vi "pre_scan_thg.vi"(6 "scan_values":dbl[](array[numeric]), 7 "override":bool, 8 "error in (no error)":errorcluster, 11 "VISA IN":refnum<visa-resource-name>) -> (0 "error out":errorcluster)   [LabVIEW 2017, in "radiant.lvlib"]
uses:
  radiant.lvlib
panel:
  out "VISA resource out":refnum<visa-resource-name>="COM9"
  in  "VISA (default)":refnum<visa-resource-name>="COM9"
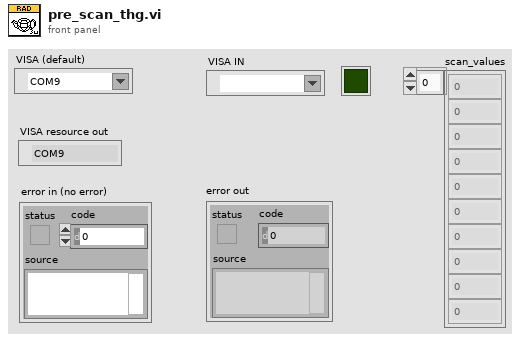
[diagram p1: front panel]
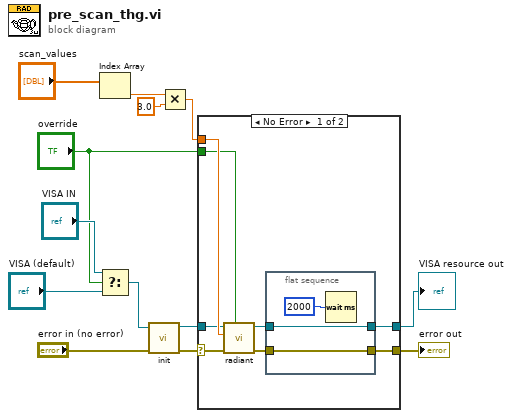
[diagram p0: block diagram]
diagram:
  n1 = Index Array(array="scan_values") -> (element=w3:dbl)  [unwired: 1 in]
  n2 = Select(t="VISA IN", s="override", f="VISA (default)") -> (s? t:f=w11:refnum<visa-resource-name>)
  n3 = call "init.vi"("error in (no error)"="error in (no error)", "VISA resource name"=w11) -> ("error out"=w9:errorcluster, "VISA resource name out"=w6:refnum<visa-resource-name>)  [unwired: 7 in, 1 out]
  n4 = Multiply(x=w3, y=3.0) -> (x*y=w1:dbl)
  n5 = case shown="No Error" w9 {
    selector: w9 -> [w21 w26]
    tunnel: [w17 w26] -> w7
    tunnel: w1 -> [w20 _]
    tunnel: w6 -> [w19 w25]
    tunnel: "override" -> [w18 _]
    tunnel: [w15 w25] -> w4
    frame No Error {
      n6 = call "radiant.vi"("override"=w18, "error in (no error)"=w21, "WL (nm)"=w20, "VISA IN"=w19) -> ("error out"=w16:errorcluster, "VISA resource out"=w14:refnum<visa-resource-name>)  [unwired: 5 in, 1 out]
      n7 = flat-sequence {
        tunnel: [w24] -> w17
        tunnel: w16 -> [w24]
        tunnel: [w22] -> w15
        tunnel: w14 -> [w22]
        frame #0 {
          n8 = Wait (ms)(milliseconds to wait=u32 2000) -> ()  [unwired: 1 out]
        }
      }
    }
    frame Error {
    }
  }
  "error out" <- w7
  "VISA resource out" <- w4
